vi "Close Ref.vi"(8 "Error In":errorcluster, 11 "DVR Ref":refnum<data-value>) -> (0 "Error Out":errorcluster)   [LabVIEW 2023, in "Arithemetic Operation.lvclass"]
doc: "The method accepts the DVR of class data as the input and closes the VI reference that the class holds."
uses:
  Arithemetic Operation.lvclass
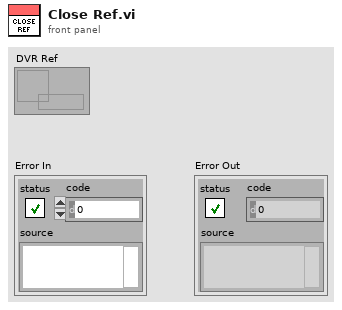
[diagram p1: front panel]
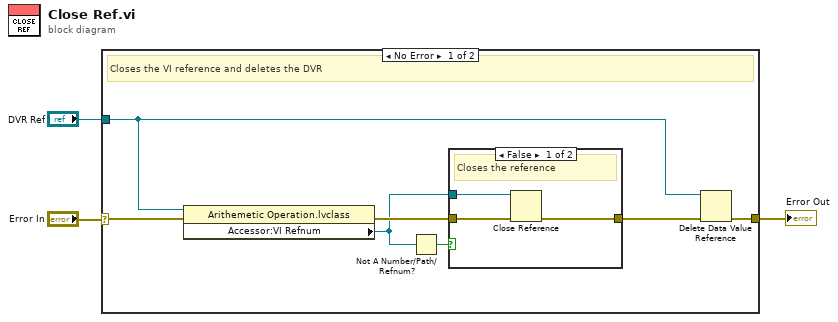
[diagram p0: block diagram]
diagram:
  n1 = case shown="No Error" "Error In" {
    selector: "Error In" -> [w7 w15]
    tunnel: "DVR Ref" -> [w5 _]
    tunnel: [w10 w15] -> w1
    frame No Error {
      # "Closes the VI reference and deletes the DVR"
      n2 = property class="Arithemetic Operation.lvclass"(reference=w5, error in=w7) -> (error out=w9:errorcluster, "Accessor:VI Refnum"=w4:refnum<vi>)  [unwired: 1 out]
      n3 = Not A Number/Path/Refnum?(number/path/refnum=w4) -> (NaN/Path/Refnum?=w8:bool)
      n4 = case shown="False" w8 {
        tunnel: w9 -> [w13 w14]
        tunnel: [w12 w14] -> w6
        tunnel: w4 -> [w11 _]
        frame False {
          # "Closes the reference"
          n5 = Close Reference(reference=w11, error in (no error)=w13) -> (error out=w12:errorcluster)
        }
        frame True {
        }
      }
      n6 = Delete Data Value Reference(data value reference=w5, error in=w6) -> (error out=w10:errorcluster)  [unwired: 1 out]
    }
    frame Error {
    }
  }
  "Error Out" <- w1
